vi "Create Message - Periodic & Trigger.vi"(7 "optional settings":T2={"Protection"=enum."None", "Enable Periodic Default"=FALSE, "Trigger Channel refnum"=18446744073709551615} {"Trigger Channel refnum" format="%x"}, 8 "error in (no error)":errorcluster, 9 "period (s)":dbl, 10 "message name":string, 11 "message group refnum in":T1=18446744073709551615 format="%.0x") -> (0 "error out":errorcluster, 2 "message refnum out":T1 format="%.0x", 3 "message group refnum out":T1 format="%.0x")   [LabVIEW 2020, in "Instrument Addon Scripting API.lvlib"]
doc: "Creates a new message section that sets the Generation Type as Periodic & Trigger. \n\nPeriodic & Trigger has the same functionality as Trigger Only but will execute the message after a set period. For example, if you set a period of 1 second and do not trigger the message, it will automatically execute after the period ends. If the message is triggered, the periodic timer resets."
uses:
  Instrument Addon Scripting API.lvlib
  TypeDefs/Message Settings.ctl
  TypeDefs/Protection Types.ctl
  <vilib>/NI VeriStand/Custom Device API/Custom Device Item Ref.ctl
  <vilib>/NI VeriStand/Custom Device API/Custom Device Channel.ctl
  <vilib>/NI VeriStand/Custom Device API/Custom Device Channel Type.ctl
  Addon/Addon Shared/Types/Message Generation Type.ctl
  <vilib>/NI VeriStand/Custom Device API/Custom Device API.lvlib
  Addon/Addon Shared/Instrument Addon Shared.lvlib
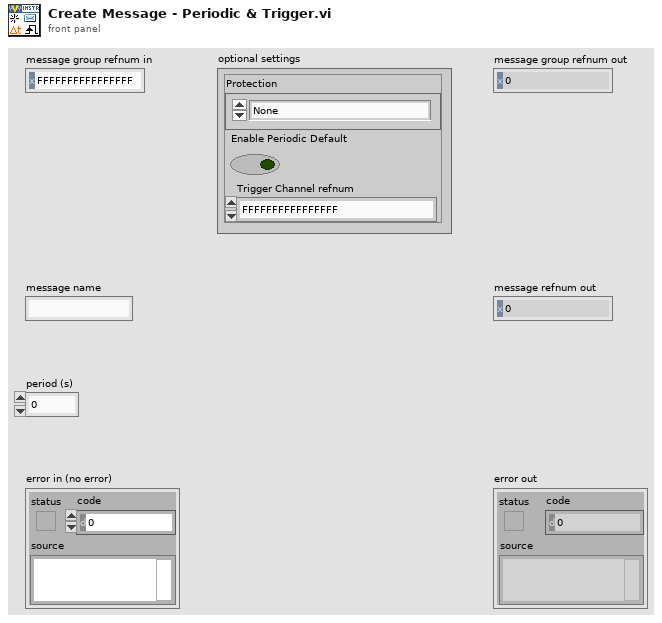
[diagram p1: front panel]
types:
  T1 = typedef "Custom Device API.lvlib/Custom Device Item Ref.ctl" = u64
  T2 = typedef "Instrument Addon Scripting API.lvlib/Message Settings.ctl" = cluster{"Protection":T3, "Enable Periodic Default":bool, "Trigger Channel refnum":u64}
  T3 = typedef "Instrument Addon Scripting API.lvlib/Protection Types.ctl" = enum16{"None", "CRC-32", "Checksum U16", "Checksum U32", "Checksum U8"}
  T4 = typedef "Instrument Addon Shared.lvlib/Message Generation Type.ctl" = enum16{"Trigger Only", "Periodic & Trigger", "Value Change & Trigger"}
  T5 = typedef "Custom Device API.lvlib/Custom Device Channel.ctl" = cluster{"Type":T6, "Units":string, "Default Value":dbl, "Faultable":bool, "Scalable":bool}
  T6 = typedef "Custom Device API.lvlib/Custom Device Channel Type.ctl" = enum16{"Input", "Output"}
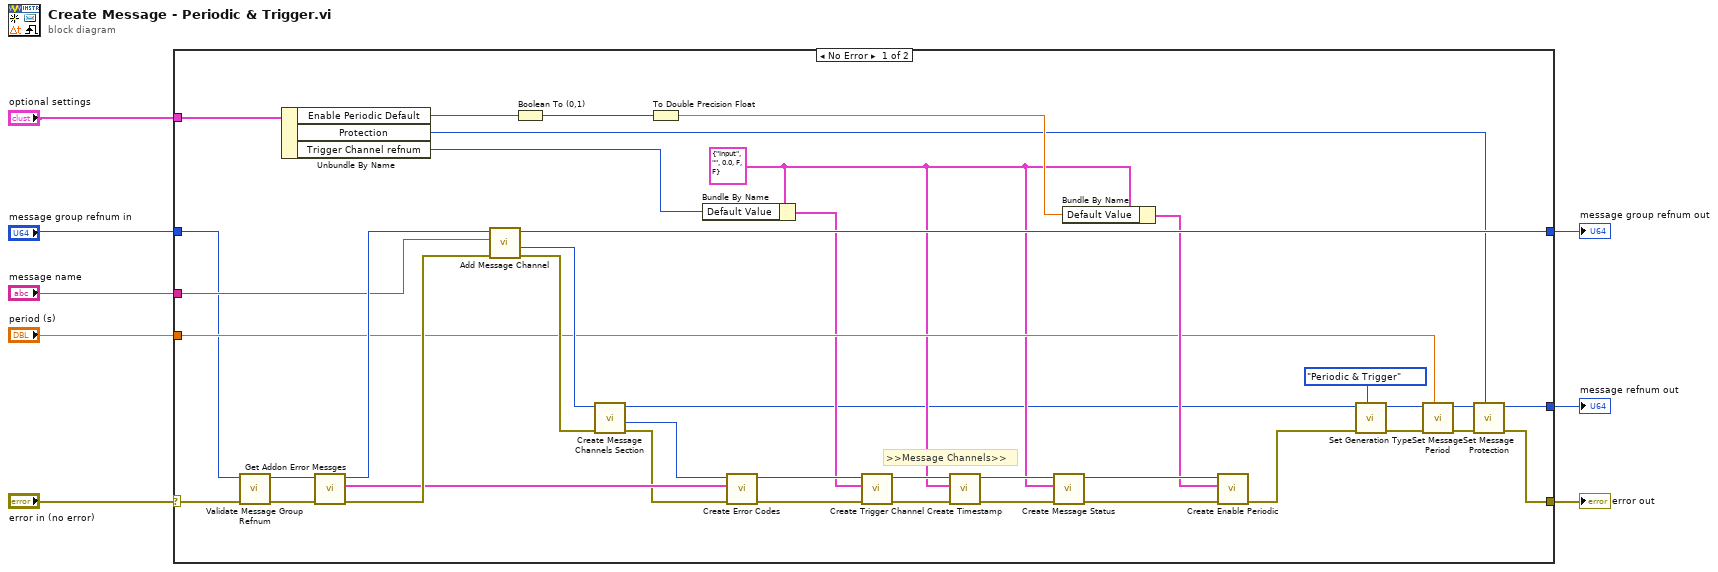
[diagram p0: block diagram]
diagram:
  n1 = case shown="No Error" "error in (no error)" {
    selector: "error in (no error)" -> [w12 w50]
    tunnel: "message group refnum in" -> [w10 w49]
    tunnel: "optional settings" -> [w43 _]
    tunnel: [w38 w49] -> w3
    tunnel: "message name" -> [w31 _]
    tunnel: "period (s)" -> [w23 _]
    tunnel: [w21 w50] -> w8
    tunnel: [w18 _] -> w2
    frame No Error {
      w17 = T5 {"Type"=enum."Input", "Units"="", "Default Value"=0.0, "Faultable"=FALSE, "Scalable"=FALSE} ("Channel")
      # ">>Message Channels>>"
      n2 = call "Validate Message Group Refnum.vi"("error in (no error)"=w12, "message group refnum in"=w10) -> ("error out"=w11:errorcluster, "message group refnum out"=w9:T1)  [unwired: 8 in]
      n3 = Unbundle By Name(w43) -> ("Enable Periodic Default"=w29:bool, "Protection"=w19:T3, "Trigger Channel refnum"=w15:u64)
      n4 = call "Get Addon Error Messges.vi"("error in (no error)"=w11, "Message Group in"=w9) -> ("error out"=w44:errorcluster, "Error Messages out"=w40:cluster{"Code":i32, "String":string}[], "Message Group out"=w39:u64)  [unwired: 7 in]
      n5 = call "Add Message Channel.vi"("error in (no error)"=w44, "Message Name"=w31, "Message Group in"=w39) -> ("error out"=w48:errorcluster, "Message out"=w41:T1, "Message Group out"=w38:T1)  [unwired: 6 in]
      n6 = Boolean To (0,1)(Boolean=w29) -> (0, 1=w28:i16)
      n7 = call "Create Message Channels Section.vi"("error in (no error)"=w48, "Message in"=w41) -> ("error out"=w37:errorcluster, "Message Channels Section out"=w36:T1, "Message out"=w13:T1)  [unwired: 7 in]
      n8 = To Double Precision Float(number=w28) -> (double precision float=w27:dbl)
      n9 = Bundle By Name(cluster=w17, "Default Value"=w15) -> (w16:T5)
      n10 = call "Create Error Codes.vi"("error in (no error)"=w37, "Error Codes"=w40, "Message Channels Section in"=w36) -> ("error out"=w34:errorcluster, "Message Channels Section out"=w35:T1)  [unwired: 7 in]
      n11 = call "Create Trigger Channel.vi"("error in (no error)"=w34, "Channel Parameters"=w16, "Message Channels Section in"=w35) -> ("error out"=w33:errorcluster, "Message Channels Section out"=w32:T1)  [unwired: 6 in, 1 out]
      n12 = call "Create Timestamp.vi"("error in (no error)"=w33, "Channel Paramters"=w17, "Message Channels Section in"=w32) -> ("error out"=w47:errorcluster, "Message Channels Section out"=w42:T1)  [unwired: 6 in, 1 out]
      n13 = call "Create Message Status.vi"("error in (no error)"=w47, "Channel Paramters"=w17, "Message Channels Section in"=w42) -> ("error out"=w46:errorcluster, "Message Channels Section out"=w45:T1)  [unwired: 7 in]
      n14 = Bundle By Name(cluster=w17, "Default Value"=w27) -> (w26:T5)
      n15 = call "Create Enable Periodic.vi"("error in (no error)"=w46, "Channel Parameters"=w26, "Message Channels Section in"=w45) -> ("error out"=w14:errorcluster)  [unwired: 7 in, 1 out]
      n16 = call "Set Generation Type.vi"("Generation Type"=Message_Generation_Type."Periodic & Trigger", "error in (no error)"=w14, "Message in"=w13) -> ("error out"=w25:errorcluster, "Message out"=w24:T1)  [unwired: 7 in]
      n17 = call "Set Message Period.vi"("Period"=w23, "error in (no error)"=w25, "Message Channel in"=w24) -> ("error out"=w22:errorcluster, "Item Ref out"=w20:T1)  [unwired: 7 in]
      n18 = call "Set Message Protection.vi"("Protection Type"=w19, "error in (no error)"=w22, "Message in"=w20) -> ("error out"=w21:errorcluster, "Message out"=w18:T1)  [unwired: 7 in]
    }
    frame Error {
    }
  }
  "error out" <- w8
  "message group refnum out" <- w3
  "message refnum out" <- w2
